vi "Polygon Intersection_Merge Points.vi"(0 "x1":dbl[](array[numeric]), 1 "left turn?":bool[](array[boolean]), 2 "index2":i32[](array[numeric]), 3 "index1":i32[](array[numeric]), 5 "y1":dbl[](array[numeric]), 7 "x2":dbl[](array[numeric]), 9 "y2":dbl[](array[numeric]), 12 "xi":dbl[](array[numeric]), 13 "yi":dbl[](array[numeric])) -> (4 "x":dbl[](array[numeric]), 6 "y":dbl[](array[numeric]))   [LabVIEW 2017, in "NI_AAL_Geometry.lvlib"]
uses:
  <vilib>/Analysis/NI_AAL_Geometry.lvlib
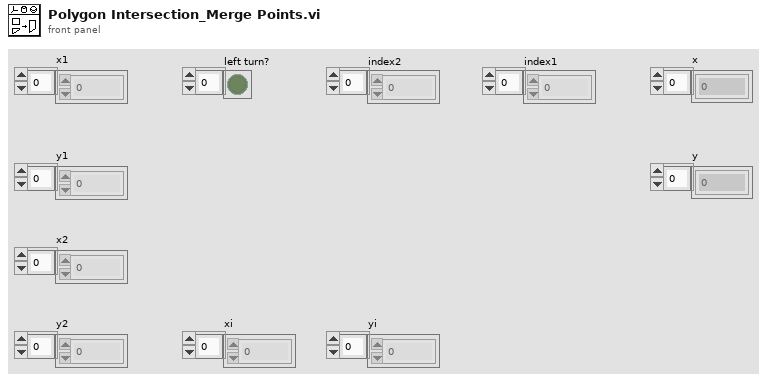
[diagram p1: front panel]
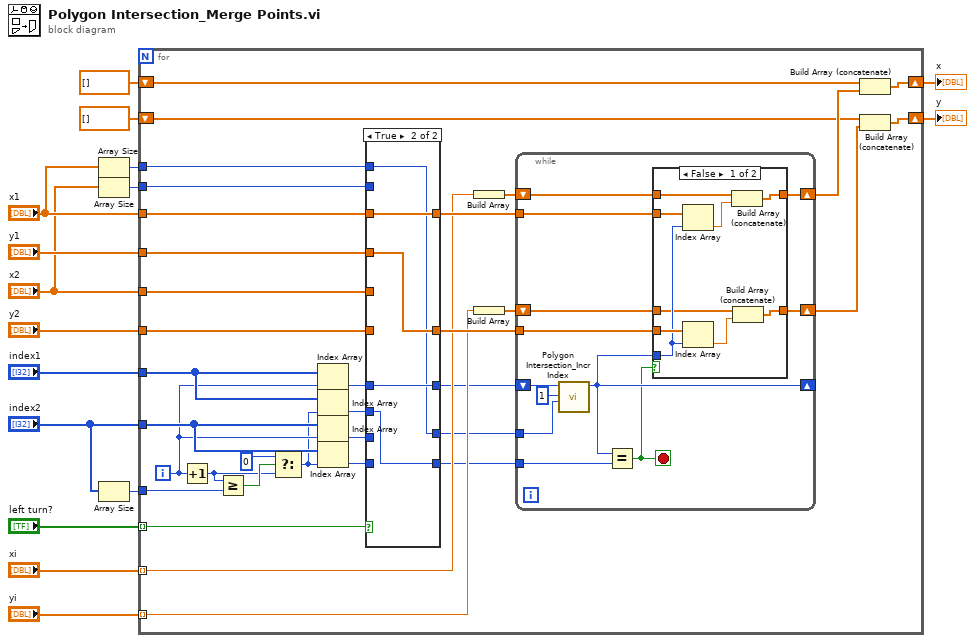
[diagram p0: block diagram]
diagram:
  n1 = Array Size(array="x1") -> (size(s)=w2:i32)
  n2 = Array Size(array="x2") -> (size(s)=w1:i32)
  n3 = Array Size(array="index2") -> (size(s)=w13:i32)
  n4 = for {
    tunnel: "left turn?" -> [w36] mode=indexing
    tunnel: "index2" -> [w49]
    tunnel: "index1" -> [w50]
    tunnel: w13 -> [w47]
    tunnel: w2 -> [w42]
    tunnel: w1 -> [w41]
    tunnel: "x1" -> [w35]
    tunnel: "y1" -> [w34]
    tunnel: "x2" -> [w33]
    tunnel: "y2" -> [w32]
    tunnel: "xi" -> [w27] mode=indexing
    tunnel: "yi" -> [w26] mode=indexing
    shift-right: [w25] -> w4
    shift-left: dbl[] [] -> [w24]
    shift-right: [w20] -> w3
    shift-left: dbl[] [] -> [w22]
    i -> [w48]
    n5 = Increment(x=w48) -> (x+1=w44:i32)
    n6 = Greater Or Equal?(x=w44, y=w47) -> (x >= y?=w46:bool)
    n7 = Select(t=0, s=w46, f=w44) -> (s? t:f=w43:i32)
    n8 = Index Array(array=w50, index=w48) -> (element=w40:i32)
    n9 = Index Array(array=w50, index=w43) -> (element=w39:i32)
    n10 = Index Array(array=w49, index=w48) -> (element=w38:i32)
    n11 = Index Array(array=w49, index=w43) -> (element=w37:i32)
    n12 = case shown="True" w36 {
      tunnel: w42 -> [_ w79]
      tunnel: w41 -> [w78 _]
      tunnel: w40 -> [_ w81]
      tunnel: w39 -> [_ w80]
      tunnel: w38 -> [w77 _]
      tunnel: w37 -> [w76 _]
      tunnel: w35 -> [_ w83]
      tunnel: w34 -> [_ w82]
      tunnel: w33 -> [w75 _]
      tunnel: w32 -> [w74 _]
      tunnel: [w75 w83] -> w31
      tunnel: [w74 w82] -> w30
      tunnel: [w77 w81] -> w19
      tunnel: [w76 w80] -> w17
      tunnel: [w78 w79] -> w18
      frame False {
      }
      frame True {
      }
    }
    n13 = Build Array(w27) -> (w29:dbl[])
    n14 = Build Array(w26) -> (w28:dbl[])
    n15 = while {
      tunnel: w17 -> [w52]
      tunnel: w18 -> [w61]
      tunnel: w31 -> [w60]
      tunnel: w30 -> [w59]
      shift-right: [w58] -> w23
      shift-left: w29 -> [w57]
      shift-right: [w56] -> w21
      shift-left: w28 -> [w55]
      shift-right: [w53] -> _
      shift-left: w19 -> [w54]
      stop <- w51 stop-if-true
      n16 = call <vilib>:"Polygon Intersection_Incr Index.vi"("polygon size"=w61, "incr"=1, "index"=w54) -> ("incr index"=w53:i32)  [unwired: 8 in]
      n17 = Equal?(x=w53, y=w52) -> (x = y?=w51:bool)
      n18 = case shown="False" w51 {
        tunnel: w60 -> [w71 _]
        tunnel: w59 -> [w70 _]
        tunnel: w53 -> [w69 _]
        tunnel: [w68 w72] -> w58
        tunnel: w57 -> [w65 w72]
        tunnel: [w67 w73] -> w56
        tunnel: w55 -> [w64 w73]
        frame False {
          n19 = Index Array(array=w71, index=w69) -> (element=w66:dbl)
          n20 = Index Array(array=w70, index=w69) -> (element=w63:dbl)
          n21 = Build Array (concatenate)(w65, w66) -> (w68:dbl[])
          n22 = Build Array (concatenate)(w64, w63) -> (w67:dbl[])
        }
        frame True {
        }
      }
    }
    n23 = Build Array (concatenate)(w24, w23) -> (w25:dbl[])
    n24 = Build Array (concatenate)(w22, w21) -> (w20:dbl[])
  }
  "x" <- w4
  "y" <- w3
